vi "Multiplier3.vi"() -> (8 "Multiplier3":refnum<class "Multiplier3.lvclass">)   [LabVIEW 2017, in "Multiplier3.lvclass"]
uses:
  Multiplier3.lvclass
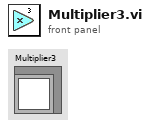
[diagram p1: front panel]
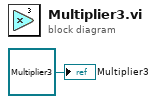
[diagram p0: block diagram]
diagram:
  "Multiplier3" <- refnum<class "Multiplier3.lvclass"> refnum ("Multiplier3.lvclass")
